vi "AllThingsColors.vi"(8 "Choice":string) -> (3 "Possible Colors":string[](array[string]))   [LabVIEW 2022 SP3]
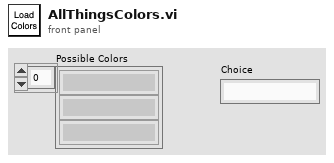
[diagram p1: front panel]
types:
  T1 = enum16{"big-endian, network order", "native, host order", "little-endian"}
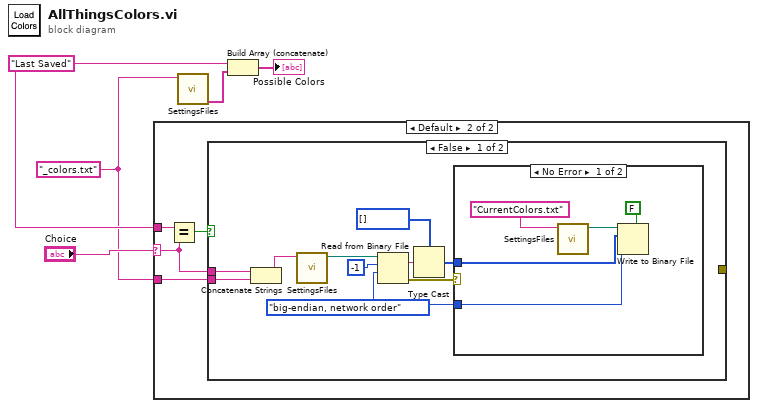
[diagram p0: block diagram]
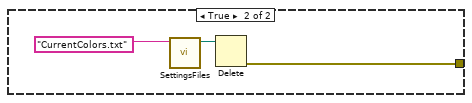
[diagram p4: hidden frame]
diagram:
  w2 = "_colors.txt" ("pattern")
  w4 = "Last Saved" ("string")
  n1 = case shown="Default" "Choice" {
    selector: "Choice" -> [_ w6]
    tunnel: w2 -> [_ w9]
    tunnel: w4 -> [_ w8]
    frame "" {
    }
    frame Default {
      n2 = Equal?(x=w8, y=w6) -> (x = y?=w7:bool)
      n3 = case shown="False" w7 {
        tunnel: w9 -> [w19 _]
        tunnel: w6 -> [w12 _]
        tunnel: [_ w27] -> _
        frame False {
          w13 = T1."big-endian, network order" ("byte order (0:big-endian, network order)")
          n4 = Concatenate Strings(w12, w19) -> (w11:string)
          n5 = call "SettingsFiles.vi"("settings file name"=w11) -> ("file path"=w10:path)  [unwired: 9 in, 1 out]
          n6 = Read from Binary File(9:w13, 10:-1 ("count (1)"), 11:w10) -> (0:w16:errorcluster, 2:w17:string)  [unwired: 3 in, 2 out]
          n7 = Type Cast(type=u32[] [] ("Color"), x=w17) -> (*(type *) &x=w14:u32[])
          n8 = case shown="No Error" w16 {
            tunnel: w14 -> [w23 _]
            tunnel: w13 -> [w22 _]
            frame No Error {
              n9 = call "SettingsFiles.vi"("settings file name"="CurrentColors.txt" ("name or relative path")) -> ("file path"=w20:path)  [unwired: 9 in, 1 out]
              n10 = Write to Binary File(file (use dialog)=w20, data=w23, 5:FALSE ("prepend array or string size? (T)"), 9:w22) -> ()  [unwired: 2 in, 3 out]
            }
            frame Error {
            }
          }
        }
        frame True {
          n11 = call "SettingsFiles.vi"("settings file name"="CurrentColors.txt" ("name or relative path")) -> ("file path"=w26:path)  [unwired: 9 in, 1 out]
          n12 = Delete(path (use dialog)=w26) -> (error out=w27:errorcluster)  [unwired: 4 in, 2 out]
        }
      }
    }
  }
  n13 = call "SettingsFiles.vi"("settings file name"=w2) -> ("filenames"=w1:string[])  [unwired: 9 in, 1 out]
  n14 = Build Array (concatenate)(w4, w1) -> (→"Possible Colors":string[])
